vi "ToCluster.vi"(8 "error in":errorcluster, 11 "Generic":refnum<class "Generic.lvclass">) -> (0 "error out":errorcluster, 3 "Cluster out":refnum<class "Cluster.lvclass">)   [LabVIEW 2014, in "Cluster.lvclass"]
uses:
  Cluster.lvclass
  Generic/Generic.lvclass
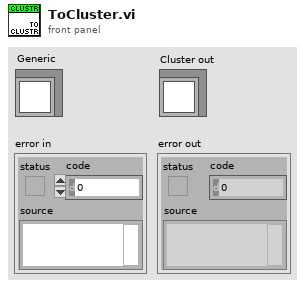
[diagram p1: front panel]
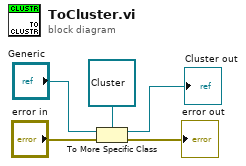
[diagram p0: block diagram]
diagram:
  n1 = To More Specific Class(target class=refnum<class "Cluster.lvclass"> refnum ("Knob in"), reference="Generic", error in="error in") -> (specific class reference=→"Cluster out":refnum<class "Cluster.lvclass">, error out=→"error out":errorcluster)
